vi "Read Paths.vi"(8 "error in (no error)":errorcluster, 11 "Tool Data in":refnum<class "Tool Data.lvclass">) -> (0 "error out":errorcluster, 2 "PathsUpdated":T1, 3 "Tool Data out":refnum<class "Tool Data.lvclass">)   [LabVIEW 2019, in "Tool Data.lvclass"]
uses:
  Tool Data.lvclass
  Settings/Path Settings/Path Settings.lvclass
  Settings/Setting Database/Typedefs/PublicEvents--Setting Database.PathsUpdated.ctl
  Settings/Setting Database/Setting Database.lvclass
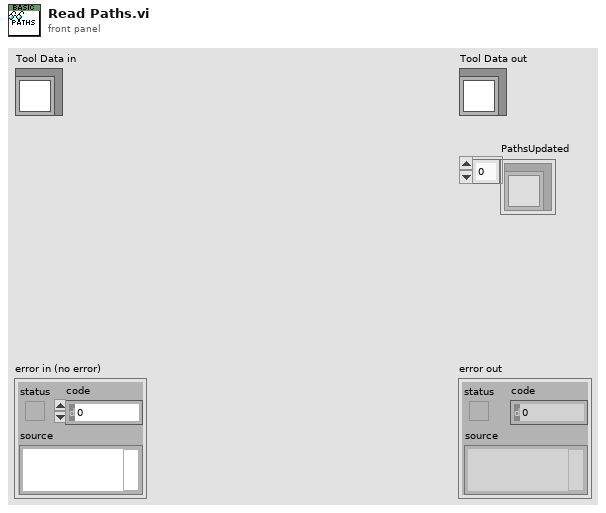
[diagram p1: front panel]
types:
  T1 = typedef "Setting Database.lvclass/PublicEvents--Setting Database.PathsUpdated.ctl" = refnum<class "Path Settings.lvclass">[]
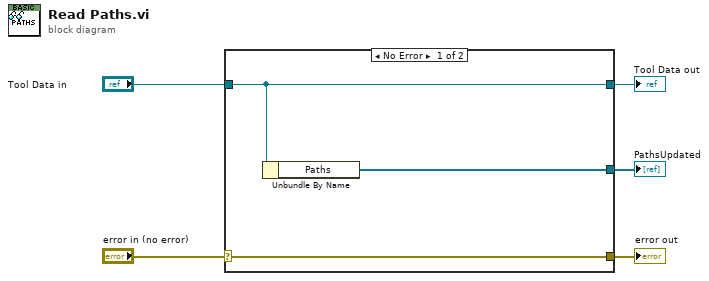
[diagram p0: block diagram]
diagram:
  n1 = case shown="No Error" "error in (no error)" {
    selector: "error in (no error)" -> [w8 w9]
    tunnel: [w8 w9] -> w4
    tunnel: [w7 w10] -> w2
    tunnel: "Tool Data in" -> [w7 w10]
    tunnel: [w6 _] -> w1
    frame No Error {
      n2 = Unbundle By Name(w7) -> ("Paths"=w6:T1)
    }
    frame Error {
    }
  }
  "error out" <- w4
  "Tool Data out" <- w2
  "PathsUpdated" <- w1
